vi "Write DCA DAC2 CMD.vi"(10 "DCA DAC2 CMD":u16, 11 "ILC in":refnum<class "ILC.lvclass">) -> (3 "ILC out":refnum<class "ILC.lvclass">)   [LabVIEW 2015, in "ILCCommon.lvlib" / "ILC.lvclass"]
uses:
  <userlib>/Common/ILC/ILC/ILC.lvclass
  <userlib>/Common/ILC/ILC/ILC.lvclass/ILC.ctl
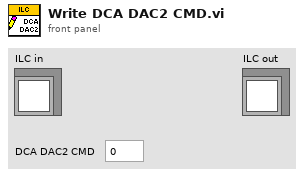
[diagram p1: front panel]
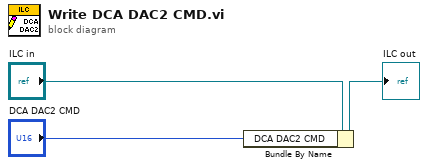
[diagram p0: block diagram]
diagram:
  n1 = Bundle By Name(cluster="ILC in", "DCA DAC2 CMD"="DCA DAC2 CMD") -> (→"ILC out":refnum<class "ILC.lvclass">)
